vi "p2.vi"() -> ()   [LabVIEW 2021, in "d5.lvlib"]
uses:
  d5.lvlib
  AOC/AOC.lvlib
panel:
  out "Answer":string
  in  "Example":string="    [D]    \n[N] [C]    \n[Z] [M] [P]\n 1   2   3 \n\nmove 1 from 2 to 1\nmove 3 from 1 to 3\nmove 2 from 2 to 1\nmove 1 from 1 to 2"
  in  "Example":bool=TRUE
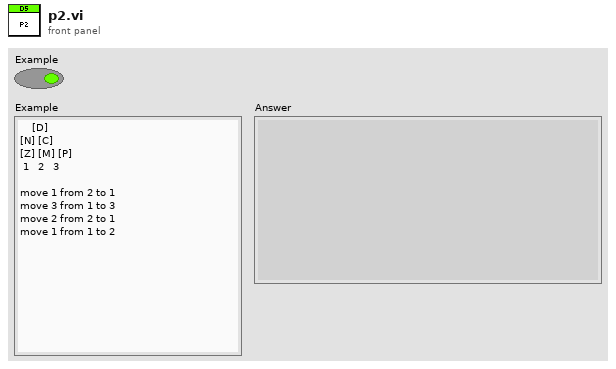
[diagram p1: front panel]
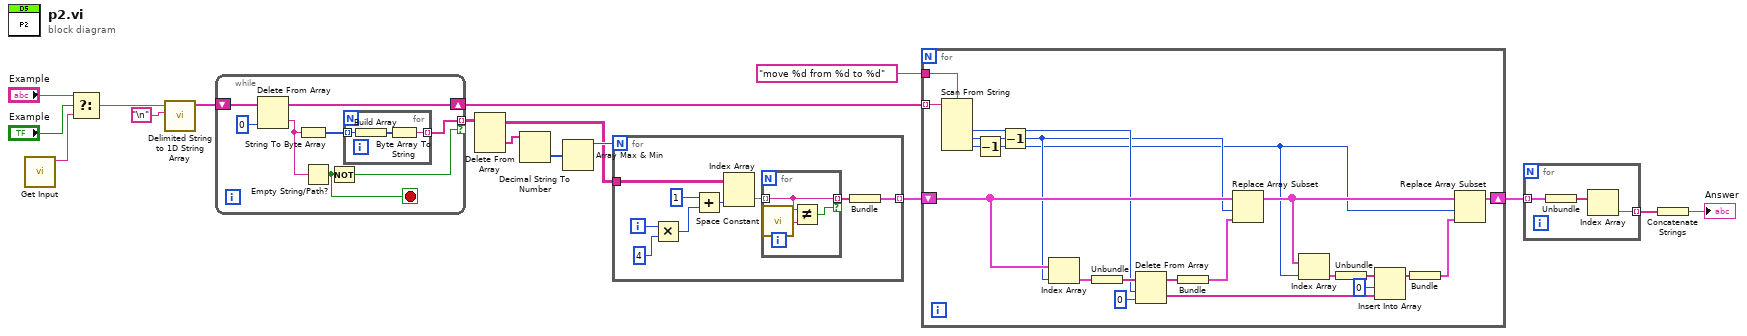
[diagram p0: block diagram]
diagram:
  n1 = call "Get Input.vi"() -> ("Input"=w17:string)  [unwired: 11 in]
  n2 = Select(t="Example", s="Example", f=w17) -> (s? t:f=w1:string)
  n3 = call <vilib>:"Delimited String to 1D String Array.vi"("delimiter"="\n", "delimited string"=w1) -> ("string array"=w13:string[])  [unwired: 9 in]
  n4 = while {
    shift-right: [w24] -> w7
    shift-left: w13 -> [w25]
    tunnel: [w18] -> w12 mode=indexing if=w22
    stop <- w21 stop-if-true
    n5 = Delete From Array(array=w25, index=0) -> (deleted portion=w20:string, array with subset deleted=w24:string[])  [unwired: 1 in]
    n6 = String To Byte Array(string=w20) -> (unsigned byte array=w19:u8[])
    n7 = Empty String/Path?(string/path=w20) -> (empty?=w21:bool)
    n8 = Not(x=w21) -> (.not. x?=w22:bool)
    n9 = for {
      tunnel: w19 -> [w28] mode=indexing
      tunnel: [w26] -> w18 mode=indexing
      n10 = Build Array(w28) -> (w27:u8[])
      n11 = Byte Array To String(unsigned byte array=w27) -> (string=w26:string)
    }
  }
  n12 = Delete From Array(array=w12) -> (deleted portion=w8:string[], array with subset deleted=w9:string[][])  [unwired: 3 in]
  n13 = Decimal String To Number(string=w8) -> (number=w11:i32[])  [unwired: 2 in, 1 out]
  n14 = Array Max & Min(array=w11) -> (max value=w10:i32)  [unwired: 3 out]
  n15 = for {
    N: w10 -> [_]
    tunnel: w9 -> [w37]
    tunnel: [w35] -> w6 mode=indexing
    i -> [w36]
    n16 = Multiply(x=w36, y=4) -> (x*y=w34:i32)
    n17 = Add(x=1, y=w34) -> (x+y=w32:i32)
    n18 = Index Array(array=w37, index (col)=w32) -> (element=w30:string[])  [unwired: 1 in]
    n19 = for {
      tunnel: w30 -> [w40] mode=indexing
      tunnel: [w40] -> w29 mode=indexing if=w39
      n20 = call <vilib>:"Space Constant.vi"() -> ("String"=w38:string)
      n21 = Not Equal?(x=w40, y=w38) -> (x != y?=w39:bool)
    }
    n22 = Bundle(w29) -> (w35:cluster{string[]})  [unwired: 1 in]
  }
  n23 = for {
    tunnel: w7 -> [w61] mode=indexing
    tunnel: "move %d from %d to %d" ("format string") -> [w60]
    shift-right: [w47] -> w4
    shift-left: w6 -> [w56]
    n24 = Scan From String(format string=w60, input string=w61) -> (output 1=w43:i32, output 2=w45:i32, output 3=w46:i32)  [unwired: 5 in, 3 out]
    n25 = Decrement(x=w46) -> (x-1=w41:i32)
    n26 = Decrement(x=w45) -> (x-1=w42:i32)
    n27 = Index Array(array=w56, index=w42) -> (element=w59:cluster{string[]})
    n28 = Unbundle(w59) -> (w58:string[])
    n29 = Delete From Array(array=w58, length=w43, index=0) -> (deleted portion=w53:string[], array with subset deleted=w55:string[])
    n30 = Bundle(w55) -> (w54:cluster{string[]})  [unwired: 1 in]
    n31 = Replace Array Subset(array=w56, new element=w54, index=w42) -> (w48:cluster{string[]}[])
    n32 = Index Array(array=w48, index=w41) -> (element=w52:cluster{string[]})
    n33 = Unbundle(w52) -> (w51:string[])
    n34 = Insert Into Array(array=w51, index=0, new element=w53) -> (w49:string[])
    n35 = Bundle(w49) -> (w44:cluster{string[]})  [unwired: 1 in]
    n36 = Replace Array Subset(array=w48, new element=w44, index=w41) -> (w47:cluster{string[]}[])
  }
  n37 = for {
    tunnel: w4 -> [w64] mode=indexing
    tunnel: [w62] -> w3 mode=indexing
    n38 = Unbundle(w64) -> (w63:string[])
    n39 = Index Array(array=w63) -> (element=w62:string)  [unwired: 1 in]
  }
  n40 = Concatenate Strings(w3) -> (→"Answer":string)
